vi "State Machine.vi"() -> ()   [LabVIEW 2010]
doc: "This VI is a template for a state machine. Just replace Process 1 and Process 2 with your states. To add more processes, modify the type defined enumerated constant. Enum order must match cluster order."
uses:
  State Enum.ctl
panel:
  in  "Menu":T1
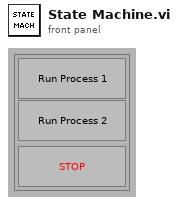
[diagram p1: front panel]
types:
  T1 = cluster{"Process 1":bool, "Process 2":bool, "stop":bool}
  T2 = typedef "State Enum.ctl" = enum32{"Idle", "Process 1", "Process 2", "Stop"}
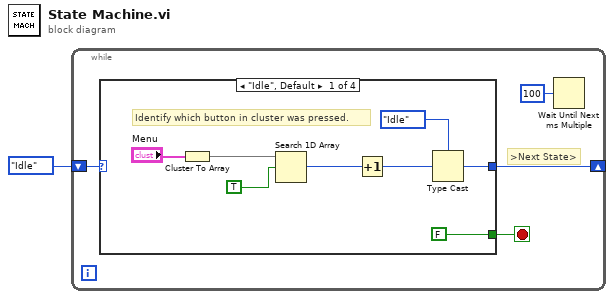
[diagram p0: block diagram]
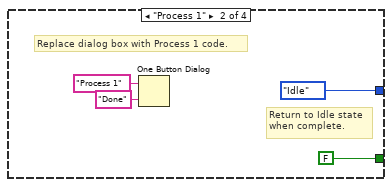
[diagram p2: hidden frame]
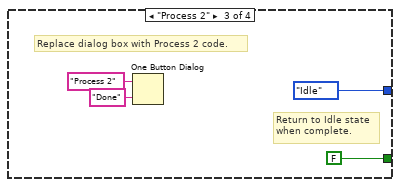
[diagram p3: hidden frame]
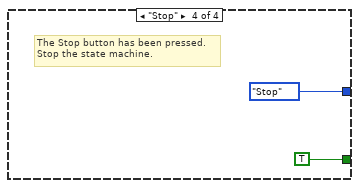
[diagram p4: hidden frame]
diagram:
  n1 = while {
    shift-right: [w4] -> _
    shift-left: State_Enum."Idle" ("Enum") -> [w5]
    stop <- w3 stop-if-true
    # ">Next State>"
    n2 = case shown="\"Idle\", Default" w5 {
      tunnel: [w10 State_Enum."Idle" ("Enum") State_Enum."Idle" ("Enum") State_Enum."Stop" ("Enum")] -> w4
      tunnel: [FALSE FALSE FALSE TRUE] -> w3
      frame "Idle", Default {
        # "Identify which button in cluster was pressed."
        n3 = Cluster To Array(cluster="Menu") -> (array=w12:bool[])
        n4 = Search 1D Array(1D array=w12, element=TRUE) -> (index of element=w7:i32)  [unwired: 1 in]
        n5 = Increment(x=w7) -> (x+1=w6:i32)
        n6 = Type Cast(type=State_Enum."Idle" ("Enum"), x=w6) -> (*(type *) &x=w10:T2)
      }
      frame "Process 1" {
        # "Return to Idle state \nwhen complete."
        # "Replace dialog box with Process 1 code."
        n7 = One Button Dialog(message="Process 1", button name ("OK")="Done") -> ()  [unwired: 1 out]
      }
      frame "Process 2" {
        # "Replace dialog box with Process 2 code."
        # "Return to Idle state \nwhen complete."
        n8 = One Button Dialog(message="Process 2", button name ("OK")="Done") -> ()  [unwired: 1 out]
      }
      frame "Stop" {
        # "The Stop button has been pressed.\nStop the state machine."
      }
    }
    n9 = Wait Until Next ms Multiple(millisecond multiple=u32 100) -> ()  [unwired: 1 out]
  }
